vi "Agilent PNA Series Config And Read Data.vi"(0 "VISA session":refnum<visa-resource-name>="GPIB0::16::INSTR", 9 "Sweep Points (801)":i32=401, 14 "Bandwidth (1000.0)":dbl=1000.0 format="%.2p") -> (4 "dup VISA session":refnum<visa-resource-name>="GPIB0::16::INSTR", 6 "Data":dbl[](array[numeric])=[-5.34917265883, -6.0051952996, -7.53487302907, -10.0389317187, -10.6485635281, -8.89561925561, -7.90396407583, -7.51160381335, -6.86207961334, -6.29267499311, -6.08245704225, -5.85167193017, -5.47711484679, -5.17463635042, -5.02839592666, -5.15941342253, -5.76240895903, -7.16671614292, -9.48193201932, -10.2000732162, -8.91799793891, -8.12700446336, -7.38779139615, -6.53229272126, -6.09092086691, -5.85659338634, -5.52800090918, -5.31752101108, -5.28721800672, -5.17374851827, -5.27656013746, -5.88261012442, -7.12184516994, -9.15323128234, -10.8028816265, -10.1688703408, -8.40413911587, -6.96518822448, -6.41535828254, -6.22147152463, -5.52087192082, -4.76290320326, -4.50807879755, -4.49011749665, -4.46059471581, -4.69867109421, -5.3387851051, -6.47704651807, -8.22820661697, -9.95331600338, -10.0946396697, -8.76961368311, -7.46488351992, -6.77474190369, -6.08350282588, -5.28148338593, -4.8177812088, -4.65798627574, -4.47297674768, -4.40275320903, -4.62796492671, -5.12716331377, -6.09626991019, -7.45499335524, -8.82710574864, -9.44663500698, -8.63373261293, -7.31451136873, -6.44919914981, -5.85972351924, -5.32641874104, -4.96347128321, -4.73027253066, -4.67739296146, -4.75628328777, -5.0140782341, -5.61671813562, -6.73535659431, -7.65162701207, -8.37023404378, -9.07118995034, -8.92129983539, -7.80992243916, -6.74299736244, -5.96107195528, -5.36078798866, -4.90868765136, -4.57614488693, -4.46793671807, -4.50444390998, -4.81802153865, -5.55467737801, -6.42960556288, -6.98011683751, -7.84763511439, -9.00214639846, -8.98116235089, -8.14033658638, -7.3195616567, -6.67528220467, -6.13245396358, -5.62747561887, -5.23353153619, -5.02771368172, -4.93637845136, -5.08364271981, -5.58277343475, -6.04359125911, -6.47341527393, -7.10597069669, -7.58630949413, -7.53457714087, -7.25497628848, -6.86815535339, -6.41153180794, -6.04120116182, -5.76011983435, -5.60300457423, -5.61321270277, -5.67018085747, -5.88754558532, -6.26307737645, -6.63853893281, -7.06285873593, -7.47997252414, -7.46328913547, -7.30301552748, -7.22474886487, -6.95119356877, -6.45685701232, -6.05117394381, -5.71070273105, -5.46128122181, -5.37411962245, -5.44352475428, -5.67839764179, -6.01476921084, -6.35749748454, -6.84757189157, -7.28984072021, -7.41593935109, -7.57461982142, -7.63185551906, -7.36859486348, -6.9535675377, -6.61380905043, -6.34847384223, -6.21217173015, -6.2057035821, -6.28260041659, -6.47807935317, -6.69162092223, -6.867356821, -7.11623327703, -7.30476753259, -7.2367457298, -7.07158545817, -6.87132098413, -6.63465343522, -6.41393979586, -6.27636114483, -6.19245894806, -6.24630892337, -6.3182419442, -6.57047330985, -6.99028453613, -7.44695583931, -7.73074384422, -7.97113333279, -8.0976688335, -8.03442531967, -7.86485562531, -7.61443889939, -7.32461998032, -7.06767680225, -6.89319765841, -6.85603142105, -6.92917031139, -7.11826903962, -7.44138480383, -7.87326223197, -8.26505067832, -8.61792838588, -8.88861714661, -8.96501047296, -8.86664443444, -8.67927686468, -8.40198016964, -8.10096915431, -7.87609860284, -7.7474441574, -7.75728803161, -7.90968997641, -8.19515479613, -8.58934282075, -9.02324180371, -9.44598034527, -9.81476607533, -10.0800060222, -10.1674746004, -10.0838140091, -9.88779008817, -9.57882234775, -9.23665271864, -8.94125331036, -8.72448352451, -8.61567717723, -8.61059757137, -8.72108436672, -8.88188181798, -9.07915397252, -9.23497742693, -9.32361810285, -9.31968605998, -9.19239133384, -8.99280452872, -8.74475232607, -8.50190654566, -8.22787529044, -8.04256200066, -7.86472901896, -7.8368329611, -7.89472170526, -8.06534732605, -8.22876869092, -8.41940937684, -8.5876208514, -8.67523968808, -8.68503716591, -8.58359634727, -8.40752390508, -8.1702692006, -7.93051259397, -7.74253058728, -7.61376590368, -7.51905158872, -7.48116673115, -7.46255151259, -7.48586042793, -7.59189750604, -7.82301015534, -8.05625594911, -8.08369943146, -8.01619135443, -7.89395617775, -7.70786618374, -7.55520979369, -7.43871322542, -7.38682812713, -7.36934687969, -7.39190379049, -7.45020091615, -7.53917859498, -7.62136263621, -7.68797878311, -7.74352709564, -7.74168025408, -7.65944114538, -7.54600554332, -7.39747879346, -7.17687737491, -7.0090847497, -6.83578128286, -6.73103686902, -6.70421964308, -6.74881836914, -6.91423553715, -7.05639628088, -7.21364747617, -7.35641250444, -7.47695672853, -7.50016197128, -7.43515852966, -7.3392918751, -7.17373509428, -6.99200514831, -6.78308761942, -6.65530841098, -6.51628635654, -6.52530634678, -6.61664604118, -6.66568311219, -6.86463370071, -7.0848338696, -7.35502521566, -7.4903683722, -7.51068460007, -7.47070211464, -7.39829592843, -7.26428770259, -7.11786132595, -7.00231119685, -6.9204280741, -6.90388171656, -6.94223028067, -7.03679020529, -7.20209301768, -7.34591105573, -7.44985976971, -7.5134130802, -7.50448312379, -7.4193769621, -7.28186229901, -7.08790700247, -6.87516659573, -6.70220400499, -6.58417329039, -6.54845934497, -6.59895698465, -6.73058270056, -6.91560687429, -7.17714579086, -7.38497379349, -7.53986055372, -7.60856904688, -7.59652946786, -7.48881004991, -7.32941649695, -7.12301143163, -6.89502648048, -6.71102356965, -6.55936199765, -6.4973066763, -6.5043684989, -6.55359778192, -6.6714673558, -6.74217386097, -6.85755213838, -6.90055086023, -6.90519574078, -6.83554775937, -6.73624373885, -6.65626653986, -6.54756504733, -6.49339041757, -6.47366475128, -6.53540935436, -6.64256811581, -6.78355920409, -6.94871116124, -7.11226649894, -7.25115352805, -7.3323408401, -7.34392090579, -7.26423415142, -7.15080726737, -7.00531057629, -6.85259154817, -6.71215368304, -6.63380897775, -6.60007989474, -6.63637656613, -6.71350512469, -6.78307367408, -6.87434133734, -6.96423845317, -7.06052879136, -7.06859446859, -7.03701424732, -7.03636522162, -7.08782110065, -7.08727310002, -7.06676565232, -7.12943675885, -7.21902115989, -7.38620438303, -7.56881608947, -7.77409964717, -7.86776348071, -7.76605845642, -7.60878394889, -7.4615458236, -7.27325620992, -6.93725178976, -6.64138368416, -6.44812031314, -6.34282764646, -6.31179534954, -6.41187151189, -6.65115346194, -7.01500660823, -7.47111238668, -7.91049259055, -8.2187696384, -8.27854665466, -8.13568525802, -7.87534307549, -7.50505904808, -7.07533898883, -6.71004305966, -6.44369431941, -6.26234801805, -6.17006203318, -6.22437893734, -6.46974122362, -6.92799765811, -7.52281454549, -8.23664604638, -9.10129135012, -9.34982748648, -9.07900361672] format="%.4f", 10 "Sweep Time":dbl=0.37501874 format="%.2p")   [LabVIEW 2018]
doc: "This VI configures the sweep parameters and reads data from the analyzer.\n\nNote: To see the data on the analyzer after running the program, from the front panel click: Trace - Math/Memory - Memory Trace"
uses:
  Agilent PNA Series/Agilent PNA Series.lvlib
panel:
  in  "Filename":path=path "E:/ff/test.lvm" caption="文件名"
  in  "CW Points":dbl=100.0
  in  "Trigger Mode (1: Continuous)":u16(ring)=2 items=["Hold", "Continuous", "Count"]
  in  "Smooth Aperture (25.0)":dbl=25.0 format="%.2p"
  in  "Smooth State":bool
  in  "CW Frq.":dbl=1000000000.0
  in  "Power Level":dbl=-10.0
  in  "Sweep Type":string(combo)="LINear"
  in  "AVG Factor":i32=5
  in  "Average?":bool
  in  "Autoscale?":bool
  in  "Format":string(combo)="MLOGarithmic"
  in  "Stop Freq (26.4 E+9)":dbl=10000000000.0 format="%.2p"
  in  "Start Freq (10.0 E+6)":dbl=5000000000.0 format="%.2p"
  out "波形图":dbl[](graph)=[-5.34917265883, -6.0051952996, -7.53487302907, -10.0389317187, -10.6485635281, -8.89561925561, -7.90396407583, -7.51160381335, -6.86207961334, -6.29267499311, -6.08245704225, -5.85167193017, -5.47711484679, -5.17463635042, -5.02839592666, -5.15941342253, -5.76240895903, -7.16671614292, -9.48193201932, -10.2000732162, -8.91799793891, -8.12700446336, -7.38779139615, -6.53229272126, -6.09092086691, -5.85659338634, -5.52800090918, -5.31752101108, -5.28721800672, -5.17374851827, -5.27656013746, -5.88261012442, -7.12184516994, -9.15323128234, -10.8028816265, -10.1688703408, -8.40413911587, -6.96518822448, -6.41535828254, -6.22147152463, -5.52087192082, -4.76290320326, -4.50807879755, -4.49011749665, -4.46059471581, -4.69867109421, -5.3387851051, -6.47704651807, -8.22820661697, -9.95331600338, -10.0946396697, -8.76961368311, -7.46488351992, -6.77474190369, -6.08350282588, -5.28148338593, -4.8177812088, -4.65798627574, -4.47297674768, -4.40275320903, -4.62796492671, -5.12716331377, -6.09626991019, -7.45499335524, -8.82710574864, -9.44663500698, -8.63373261293, -7.31451136873, -6.44919914981, -5.85972351924, -5.32641874104, -4.96347128321, -4.73027253066, -4.67739296146, -4.75628328777, -5.0140782341, -5.61671813562, -6.73535659431, -7.65162701207, -8.37023404378, -9.07118995034, -8.92129983539, -7.80992243916, -6.74299736244, -5.96107195528, -5.36078798866, -4.90868765136, -4.57614488693, -4.46793671807, -4.50444390998, -4.81802153865, -5.55467737801, -6.42960556288, -6.98011683751, -7.84763511439, -9.00214639846, -8.98116235089, -8.14033658638, -7.3195616567, -6.67528220467, -6.13245396358, -5.62747561887, -5.23353153619, -5.02771368172, -4.93637845136, -5.08364271981, -5.58277343475, -6.04359125911, -6.47341527393, -7.10597069669, -7.58630949413, -7.53457714087, -7.25497628848, -6.86815535339, -6.41153180794, -6.04120116182, -5.76011983435, -5.60300457423, -5.61321270277, -5.67018085747, -5.88754558532, -6.26307737645, -6.63853893281, -7.06285873593, -7.47997252414, -7.46328913547, -7.30301552748, -7.22474886487, -6.95119356877, -6.45685701232, -6.05117394381, -5.71070273105, -5.46128122181, -5.37411962245, -5.44352475428, -5.67839764179, -6.01476921084, -6.35749748454, -6.84757189157, -7.28984072021, -7.41593935109, -7.57461982142, -7.63185551906, -7.36859486348, -6.9535675377, -6.61380905043, -6.34847384223, -6.21217173015, -6.2057035821, -6.28260041659, -6.47807935317, -6.69162092223, -6.867356821, -7.11623327703, -7.30476753259, -7.2367457298, -7.07158545817, -6.87132098413, -6.63465343522, -6.41393979586, -6.27636114483, -6.19245894806, -6.24630892337, -6.3182419442, -6.57047330985, -6.99028453613, -7.44695583931, -7.73074384422, -7.97113333279, -8.0976688335, -8.03442531967, -7.86485562531, -7.61443889939, -7.32461998032, -7.06767680225, -6.89319765841, -6.85603142105, -6.92917031139, -7.11826903962, -7.44138480383, -7.87326223197, -8.26505067832, -8.61792838588, -8.88861714661, -8.96501047296, -8.86664443444, -8.67927686468, -8.40198016964, -8.10096915431, -7.87609860284, -7.7474441574, -7.75728803161, -7.90968997641, -8.19515479613, -8.58934282075, -9.02324180371, -9.44598034527, -9.81476607533, -10.0800060222, -10.1674746004, -10.0838140091, -9.88779008817, -9.57882234775, -9.23665271864, -8.94125331036, -8.72448352451, -8.61567717723, -8.61059757137, -8.72108436672, -8.88188181798, -9.07915397252, -9.23497742693, -9.32361810285, -9.31968605998, -9.19239133384, -8.99280452872, -8.74475232607, -8.50190654566, -8.22787529044, -8.04256200066, -7.86472901896, -7.8368329611, -7.89472170526, -8.06534732605, -8.22876869092, -8.41940937684, -8.5876208514, -8.67523968808, -8.68503716591, -8.58359634727, -8.40752390508, -8.1702692006, -7.93051259397, -7.74253058728, -7.61376590368, -7.51905158872, -7.48116673115, -7.46255151259, -7.48586042793, -7.59189750604, -7.82301015534, -8.05625594911, -8.08369943146, -8.01619135443, -7.89395617775, -7.70786618374, -7.55520979369, -7.43871322542, -7.38682812713, -7.36934687969, -7.39190379049, -7.45020091615, -7.53917859498, -7.62136263621, -7.68797878311, -7.74352709564, -7.74168025408, -7.65944114538, -7.54600554332, -7.39747879346, -7.17687737491, -7.0090847497, -6.83578128286, -6.73103686902, -6.70421964308, -6.74881836914, -6.91423553715, -7.05639628088, -7.21364747617, -7.35641250444, -7.47695672853, -7.50016197128, -7.43515852966, -7.3392918751, -7.17373509428, -6.99200514831, -6.78308761942, -6.65530841098, -6.51628635654, -6.52530634678, -6.61664604118, -6.66568311219, -6.86463370071, -7.0848338696, -7.35502521566, -7.4903683722, -7.51068460007, -7.47070211464, -7.39829592843, -7.26428770259, -7.11786132595, -7.00231119685, -6.9204280741, -6.90388171656, -6.94223028067, -7.03679020529, -7.20209301768, -7.34591105573, -7.44985976971, -7.5134130802, -7.50448312379, -7.4193769621, -7.28186229901, -7.08790700247, -6.87516659573, -6.70220400499, -6.58417329039, -6.54845934497, -6.59895698465, -6.73058270056, -6.91560687429, -7.17714579086, -7.38497379349, -7.53986055372, -7.60856904688, -7.59652946786, -7.48881004991, -7.32941649695, -7.12301143163, -6.89502648048, -6.71102356965, -6.55936199765, -6.4973066763, -6.5043684989, -6.55359778192, -6.6714673558, -6.74217386097, -6.85755213838, -6.90055086023, -6.90519574078, -6.83554775937, -6.73624373885, -6.65626653986, -6.54756504733, -6.49339041757, -6.47366475128, -6.53540935436, -6.64256811581, -6.78355920409, -6.94871116124, -7.11226649894, -7.25115352805, -7.3323408401, -7.34392090579, -7.26423415142, -7.15080726737, -7.00531057629, -6.85259154817, -6.71215368304, -6.63380897775, -6.60007989474, -6.63637656613, -6.71350512469, -6.78307367408, -6.87434133734, -6.96423845317, -7.06052879136, -7.06859446859, -7.03701424732, -7.03636522162, -7.08782110065, -7.08727310002, -7.06676565232, -7.12943675885, -7.21902115989, -7.38620438303, -7.56881608947, -7.77409964717, -7.86776348071, -7.76605845642, -7.60878394889, -7.4615458236, -7.27325620992, -6.93725178976, -6.64138368416, -6.44812031314, -6.34282764646, -6.31179534954, -6.41187151189, -6.65115346194, -7.01500660823, -7.47111238668, -7.91049259055, -8.2187696384, -8.27854665466, -8.13568525802, -7.87534307549, -7.50505904808, -7.07533898883, -6.71004305966, -6.44369431941, -6.26234801805, -6.17006203318, -6.22437893734, -6.46974122362, -6.92799765811, -7.52281454549, -8.23664604638, -9.10129135012, -9.34982748648, -9.07900361672]
  in  "Measurement Name (MY_MEAS)":string="MY_MEAS"
  in  "Measurement Type (0: S11)":i32(ring)=2 items=["S11", "S12", "S21", "S22", "A", "B", "R1", "R2", "A/B", "B/A"]
  # "(c) 2005-2015 National Instruments.  ALL RIGHTS RESERVED."
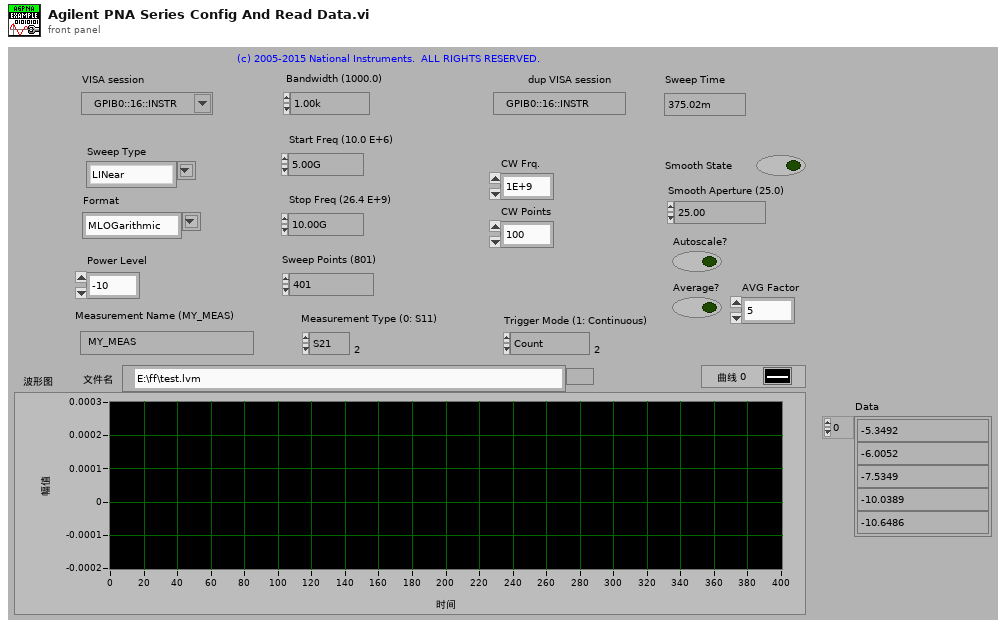
[diagram p1: front panel]
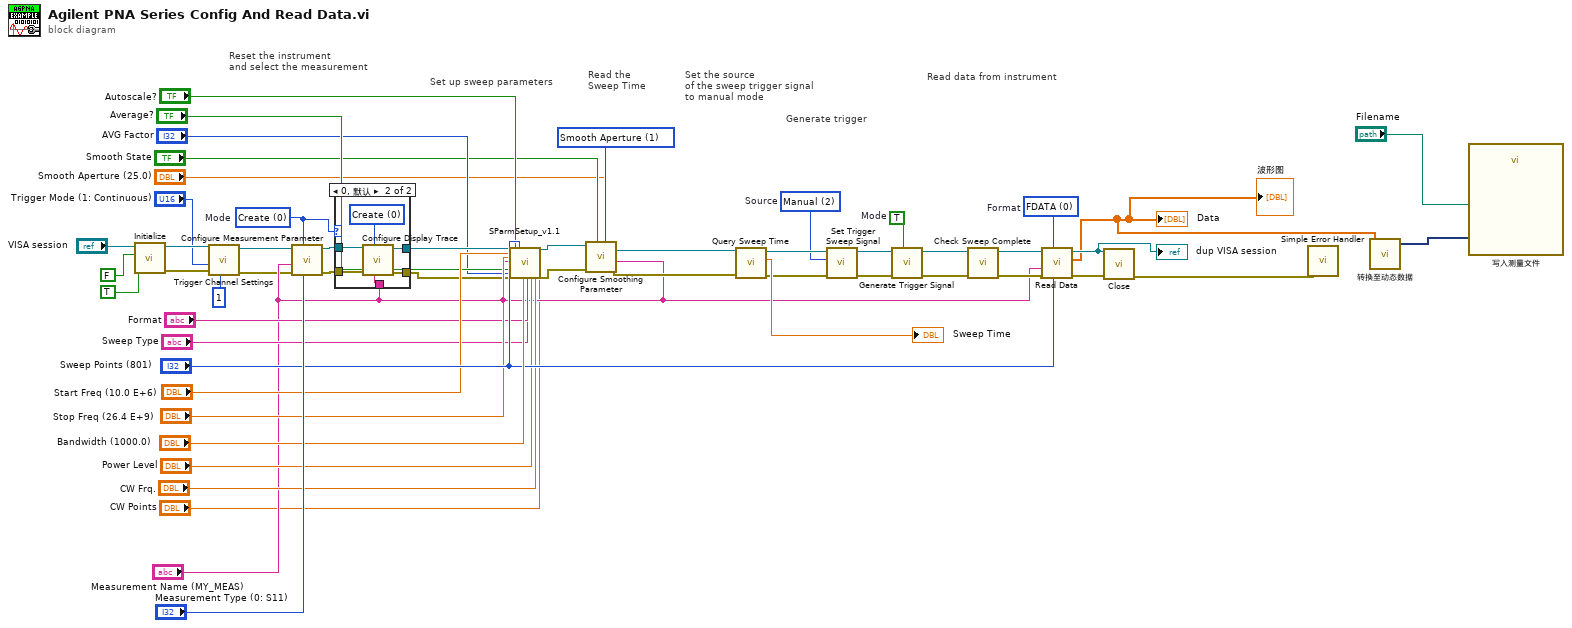
[diagram p0: block diagram]
diagram:
  w12 = u16 1 items=["Smooth Points", "Smooth Aperture"] ("Mode (0: Smooth Points)")
  w41 = TRUE  # Mode
  w42 = u16 2 items=["Immediate", "External", "Manual"]  # Source
  w33 = u16 0 items=["Create", "Delete", "Select"]  # Mode
  w53 = u16 0 items=["FDATA", "SDATA", "FMEM", "SMEM", "SDIV"]  # Format
  # "Generate trigger"
  # "Read the \nSweep Time"
  # "Set up sweep parameters"
  # "Read data from instrument"
  # "Set the source \nof the sweep trigger signal \nto manual mode"
  # "Reset the instrument\nand select the measurement"
  n1 = call "Initialize.vi"("Reset (T: Reset)"=TRUE, "ID Query (T: Check)"=FALSE, "Instrument Resource Name"="VISA session") -> ("error out"=w9:errorcluster, "dup VISA session"=w10:refnum<visa-resource-name>)  [unwired: 7 in]
  n2 = call "Trigger Channel Settings.vi"("Trigger Count (1)"=1, "Error In (no error)"=w9, "Trigger Mode (1: Continuous)"="Trigger Mode (1: Continuous)", "VISA session"=w10) -> ("Error Out"=w8:errorcluster, "dup VISA session"=w7:refnum<visa-resource-name>)  [unwired: 6 in]
  n3 = call "Configure Measurement Parameter.vi"("Measurement Type (0: S11)"="Measurement Type (0: S11)", "Mode (0: Create)"=w33, "Error In (no error)"=w8, "Measurement Name (MY_MEAS)"="Measurement Name (MY_MEAS)", "VISA Resource Name"=w7) -> ("Error Out"=w35:errorcluster, "VISA Resource Name Out"=w36:refnum<visa-resource-name>)  [unwired: 5 in]
  n4 = case shown="0, 默认" w33 {
    tunnel: w36 -> [w55 w61]
    tunnel: [w55 w60] -> w26
    tunnel: w35 -> [w54 w59]
    tunnel: [w54 w58] -> w27
    tunnel: "Measurement Name (MY_MEAS)" -> [_ w56]
    frame 2 {
    }
    frame 0, Default {
      w57 = u16 0 items=["Create", "Delete"] ("Mode (0: Create)")
      n5 = call "Configure Display Trace.vi"("Measurement Name (MY_MEAS)"=w56, "Mode (0: Create)"=w57, "Error In (no error)"=w59, "VISA Resource Name"=w61) -> ("Error Out"=w58:errorcluster, "VISA Resource Name Out"=w60:refnum<visa-resource-name>)  [unwired: 6 in]
    }
  }
  n6 = call "SParmSetup_v1.1.vi"("VISA IN"=w26, "Start Frequency"="Start Freq (10.0 E+6)", "Stop Frequency"="Stop Freq (26.4 E+9)", "Filename"="Measurement Name (MY_MEAS)", "Average?"="Average?", "AVG Factor"="AVG Factor", "error in"=w27, "Autoscale?"="Autoscale?", "Points"="Sweep Points (801)", "IF BW"="Bandwidth (1000.0)", "Format"="Format", "Sweep Type"="Sweep Type", "Power Level"="Power Level", "CW Frq."="CW Frq.", "CW Points"="CW Points") -> ("VISA Out"=w18:refnum<visa-resource-name>, "error out"=w16:errorcluster)  [unwired: 11 in]
  n7 = call "Configure Smoothing Parameter.vi"("Smooth Aperture (25.0)"="Smooth Aperture (25.0)", "Mode (0: Smooth Points)"=w12, "Smooth State (F: Off)"="Smooth State", "Error In (no error)"=w16, "Measurement Name (MY_MEAS)"="Measurement Name (MY_MEAS)", "VISA Resource Name"=w18) -> ("Error Out"=w15:errorcluster, "VISA Resource Name Out"=w17:refnum<visa-resource-name>)  [unwired: 4 in]
  n8 = call "Query Sweep Time.vi"("Error In (no error)"=w15, "VISA Resource Name"=w17) -> ("Error Out"=w43:errorcluster, "Sweep Time"=→"Sweep Time":dbl, "VISA Resource Name Out"=w44:refnum<visa-resource-name>)  [unwired: 7 in]
  n9 = call "Set Trigger Sweep Signal.vi"("Error In (no error)"=w43, "Source (0: Immediate)"=w42, "VISA session"=w44) -> ("Error Out"=w51:errorcluster, "dup VISA session"=w50:refnum<visa-resource-name>)  [unwired: 7 in]
  n10 = call "Generate Trigger Signal.vi"("Mode (T: Initiate)"=w41, "Error In (no error)"=w51, "VISA Resource Name"=w50) -> ("Error Out"=w47:errorcluster, "VISA Resource Name Out"=w48:refnum<visa-resource-name>)  [unwired: 7 in]
  n11 = call "Check Sweep Complete.vi"("Error In (no error)"=w47, "VISA Resource Name"=w48) -> ("Error Out"=w45:errorcluster, "VISA Resource Name Out"=w46:refnum<visa-resource-name>)  [unwired: 7 in, 1 out]
  n12 = call "Read Data.vi"("Sample Count (401)"="Sweep Points (801)", "Format  (0: FDATA)"=w53, "Error In (no error)"=w45, "Measurement Name (MY_MEAS)"="Measurement Name (MY_MEAS)", "VISA Resource Name"=w46) -> ("Error Out"=w40:errorcluster, "Data"=w3:dbl[], "VISA Resource Name Out"=w34:refnum<visa-resource-name>)  [unwired: 4 in]
  "dup VISA session" <- w34
  "Data" <- w3
  "波形图" <- w3
  n13 = call "Close.vi"("Error In (no error)"=w40, "VISA Resource Name"=w34) -> ("Error Out"=w39:errorcluster)  [unwired: 9 in]
  n14 = call <vilib>:"Simple Error Handler.vi"("error in (no error)"=w39) -> ()  [unwired: 4 in, 5 out]
  n15 = call "转换至动态数据"("Array"=w3) -> ("Dynamic Data Type"=w2:dynamicdata)  [unwired: 3 in]
  n16 = call "写入测量文件"("Signals"=w2, "Filename"="Filename") -> ()  [unwired: 15 in, 3 out]
